vi "Set AsyncCommandQ ref.vi"(10 "AsyncCommandQ":refnum<queue>, 11 "TimerDRV in":refnum<class "TimerDRV.lvclass">) -> (3 "TimerDRV out":refnum<class "TimerDRV.lvclass">)   [LabVIEW 2019, in "TimingDRV Engine.lvlib" / "TimerDRV.lvclass"]
uses:
  TimerDRV.lvclass
  TypeDefs/Command Package.ctl
  TypeDefs/Command.ctl
  TimerDRV.lvclass/TimerDRV.ctl
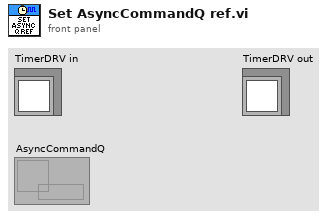
[diagram p1: front panel]
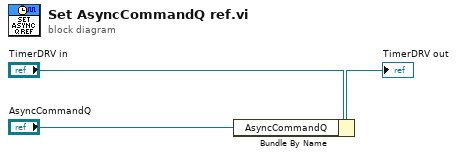
[diagram p0: block diagram]
diagram:
  n1 = Bundle By Name(cluster="TimerDRV in", "AsyncCommandQ"="AsyncCommandQ") -> (→"TimerDRV out":refnum<class "TimerDRV.lvclass">)
